vi "niScope Cal Self Calibrate.vi"(0 "instrument handle":refnum<k15>, 5 "channels":string, 9 "Option":T1 items=["Self Calibrate All Channels", "Restore External Calibration"], 11 "error in":errorcluster) -> (4 "instrument handle out":refnum<k15>, 15 "error out":errorcluster)   [LabVIEW 2013]
doc: "Self-calibrates most NI digitizers, including all SMC-based devices and most Traditional NI-DAQ (Legacy) devices."
uses:
  <instrlib>/niScope/Controls/niScope self cal option.ctl
  niScope_32.dll
panel:
  # "Note: disconnect or disable AC input signals before running.\nCalibration may take several minutes."
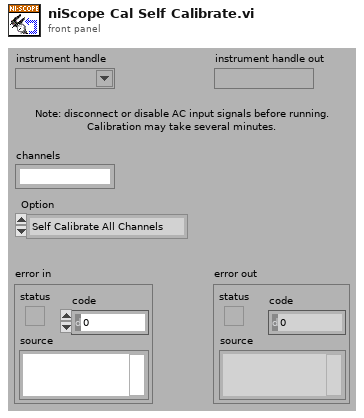
[diagram p1: front panel]
types:
  T1 = typedef "niScope self cal option.ctl" = i32
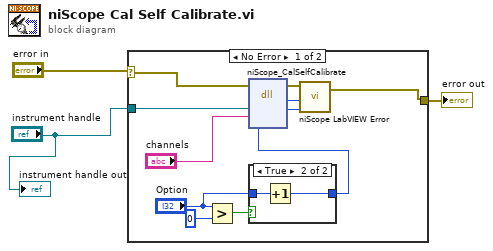
[diagram p0: block diagram]
diagram:
  n1 = case shown="No Error" "error in" {
    selector: "error in" -> [w4 w17]
    tunnel: [w5 w17] -> w3
    tunnel: "instrument handle" -> [w13 _]
    frame No Error {
      n2 = Greater?(x="Option", y=0) -> (0:w8:bool)
      n3 = case shown="True" w8 {
        tunnel: [w14 w16] -> w10
        tunnel: "Option" -> [w14 w15]
        frame False {
        }
        frame True {
          n4 = Increment(x=w15) -> (x+1=w16:T1)
        }
      }
      n5 = dll-call lib="niScope_*.*" fn="niScope_CalSelfCalibrate"("instrument handle"=w13, "Channel Name"="channels", "Options"=w10) -> ("status"=w6:i32, "instrument handle"=w7:u32)  [unwired: 5 in, 2 out]
      n6 = call <instrlib>:"niScope LabVIEW Error.vi"("instrument handle"=w7, "niScope error code (0)"=w6, "error in (no error)"=w4) -> ("error out"=w5:errorcluster)  [unwired: 2 in]
    }
    frame Error {
    }
  }
  "error out" <- w3
  "instrument handle out" <- "instrument handle"
